vi "Write Unit label.vi"(5 "Unit label":refnum<class "Text.lvclass">, 9 "GraphScale in":refnum<class "GraphScale.lvclass">) -> (3 "GraphScale out":refnum<class "GraphScale.lvclass">)   [LabVIEW 2014, in "GraphScale.lvclass"]
uses:
  GraphScale.lvclass
  Text/Text.lvclass
  GraphScale.lvclass/GraphScale.ctl
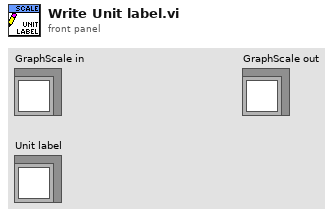
[diagram p1: front panel]
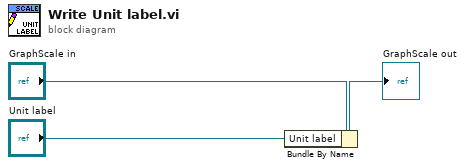
[diagram p0: block diagram]
diagram:
  n1 = Bundle By Name(cluster="GraphScale in", "Unit label"="Unit label") -> (→"GraphScale out":refnum<class "GraphScale.lvclass">)
